vi "TX_base_signal.vi"(6 "reset":bool, 7 "code":enum16{"无编码", "RS码", "卷积码"}(ring), 8 "error in (no error)":errorcluster, 9 "symbol rate (Hz)":dbl=1.0 format="%.2f", 10 "pulse shaping samples per symbol (16)":i32=16, 11 "输入要传输的信息":string="hello,my name is liuxiaowei") -> (0 "error out":errorcluster, 1 "system_message":T1, 3 "output complex waveform":T2 {"Y" format="%.3f"; "dt" format="%^.2e"; "t0" format="%.4f"})   [LabVIEW 2010]
uses:
  <vilib>/addons/Modulation/Analog/controls/Complex Data Waveform.ctl
  <vilib>/AddOns/Modulation/Digital/General/MT Generate MSK System Parameters.vi
  <vilib>/AddOns/Modulation/Digital/General/MT Map Bits to MSK symbols.vi
  <vilib>/addons/Modulation/niDMT.lvlib
  <vilib>/addons/Modulation/niAMT.lvlib
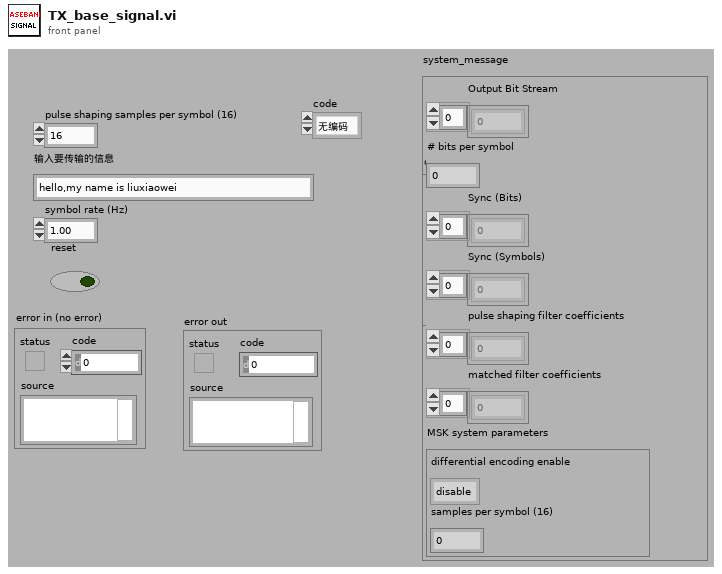
[diagram p1: front panel]
types:
  T1 = cluster{"Output Bit Stream":i8[], "# bits per symbol":i32, "Sync (Bits)":i8[], "Sync (Symbols)":cdb[], "pulse shaping filter coefficients":dbl[], "matched filter coefficients":dbl[], "MSK system parameters":cluster{"differential encoding enable":enum16{"disable", "enable"}, "samples per symbol (16)":i32}}
  T2 = typedef "niAMT.lvlib/Complex Data Waveform.ctl" = cluster{"t0":dbl, "dt":dbl, "Y":cdb[]}
  T3 = enum16{"FSK", "PSK", "QAM", "MSK", "PAM", "ASK", "CPM"}
  T4 = enum16{"none", "Raised Cosine", "Root Raised Cos", "Gaussian"}
  T5 = cluster{"differential encoding enable":enum16{"disable", "enable"}, "samples per symbol (16)":i32}
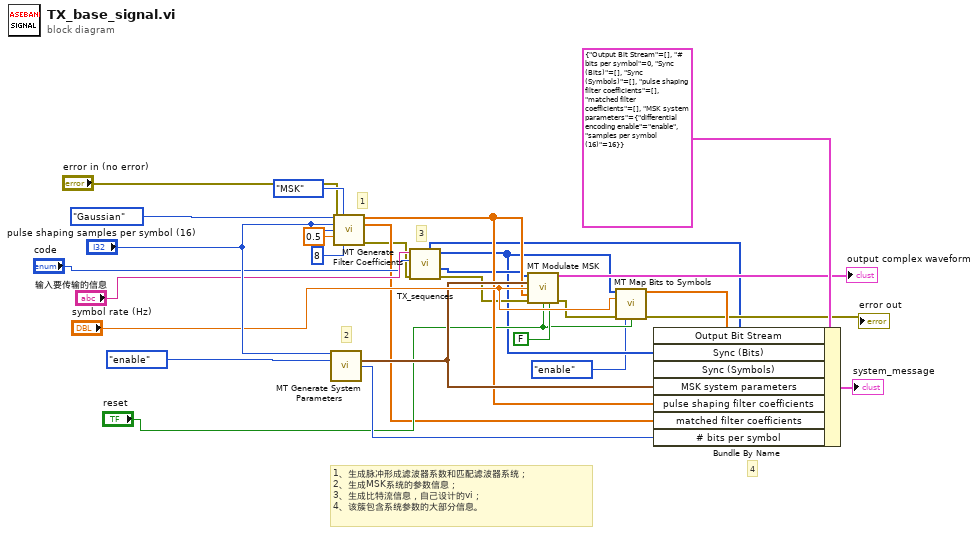
[diagram p0: block diagram]
diagram:
  # "1、生成脉冲形成滤波器系数和匹配滤波器系统；\n2、生成MSK系统的参数信息；\n3、生成比特流信息，自己设计的vi；\n4、该簇包含系统参数的大部分信息。"
  # "4"
  # "3"
  # "2"
  # "1"
  n1 = call-poly <vilib>:"MT Generate System Parameters.vi"("samples per symbol (16)"="pulse shaping samples per symbol (16)", "differential encoding enable"=enum16{"disable", "enable"}."enable") -> ("MSK system parameters"=w20:T5, "bits per symbol"=w18:i32)  [unwired: 11 in, 1 out]
  n2 = call <vilib>:"MT Generate Filter Coefficients.vi"("pulse shaping filter (none)"=T4."Gaussian", "modulation type"=T3."MSK", "pulse shaping samples per symbol (16)"="pulse shaping samples per symbol (16)", "matched samples per symbol (16)"="pulse shaping samples per symbol (16)", "filter parameter"=0.5, "error in (no error)"="error in (no error)", "filter length (symbols)"=8) -> ("pulse shaping filter coefficients"=w19:dbl[], "matched filter coefficients"=w7:dbl[], "error out"=w6:errorcluster)  [unwired: 6 in]
  n3 = call "TX_sequences.vi"("error in (no error)"=w6, "code"="code", "输入要传输的信息"="输入要传输的信息") -> ("signal for calculate ber"=w3:i8[], "error out"=w5:errorcluster, "message_bit"=w4:i8[], "syc bit"=w2:i8[])  [unwired: 3 in, 1 out]
  n4 = call <vilib>:"MT Modulate MSK.vi"("input bit stream"=w4, "MSK system parameters"=w20, "symbol rate (Hz)"="symbol rate (Hz)", "pulse shaping filter coefficients"=w19, "error in (no error)"=w5, "reset? (T)"="reset", "flush buffers? (F)"=FALSE) -> ("output complex waveform"=→"output complex waveform":T2, "error out"=w22:errorcluster)  [unwired: 6 in, 1 out]
  n5 = call-poly <vilib>:"MT Map Bits to Symbols.vi"("input bit stream"=w2, "symbol rate, Hz"="symbol rate (Hz)", "error in (no error)"=w22, "differential encoding enable"=enum16{"disable", "enable"}."enable", "reset? (T)"="reset") -> ("symbols"=w21:dbl[], "error out"=→"error out":errorcluster)  [unwired: 9 in]
  n6 = Bundle By Name(cluster=T1 {"Output Bit Stream"=[], "# bits per symbol"=0, "Sync (Bits)"=[], "Sync (Symbols)"=[], "pulse shaping filter coefficients"=[], "matched filter coefficients"=[], "MSK system parameters"={"differential encoding enable"=enum."enable", "samples per symbol (16)"=16}} ("Signal Description"), "Output Bit Stream"=w3, "Sync (Bits)"=w2, "Sync (Symbols)"=w21, "MSK system parameters"=w20, "pulse shaping filter coefficients"=w19, "matched filter coefficients"=w7, "# bits per symbol"=w18) -> (→"system_message":T1)
